vi "Deinitialize Cameras.vi"(8 "error in":errorcluster, 11 "Gantry in":refnum<class "Gantry.lvclass">) -> (0 "error out":errorcluster, 3 "Gantry out":refnum<class "Gantry.lvclass">)   [LabVIEW 2017, in "Gantry.lvclass"]
uses:
  Gantry.lvclass
  FlexWorktable/FlexWorktable.lvclass
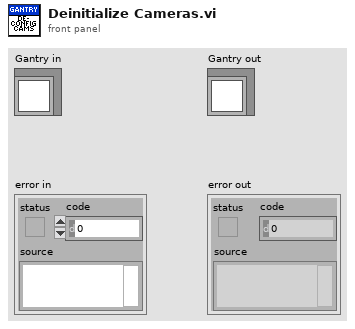
[diagram p1: front panel]
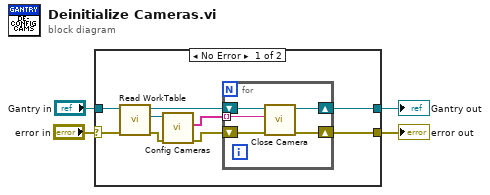
[diagram p0: block diagram]
diagram:
  n1 = case shown="No Error" "error in" {
    selector: "error in" -> [w10 w20]
    tunnel: [w12 w20] -> w3
    tunnel: [w13 w19] -> w1
    tunnel: "Gantry in" -> [w11 w19]
    frame No Error {
      n2 = call-dynamic "Read WorkTable.vi"("error in"=w10, "Gantry Class in"=w11) -> ("error out"=w7:errorcluster, "Worktable"=w9:refnum<class "FlexWorktable.lvclass">, "Gantry Class out"=w8:refnum<class "Gantry.lvclass">)  [unwired: 7 in]
      n3 = call "Config Cameras.vi"("error in (no error)"=w7, "FlexWorktable in"=w9) -> ("error out"=w5:errorcluster, "Array"=w6:string[])  [unwired: 7 in, 1 out]
      n4 = for {
        tunnel: w6 -> [w18] mode=indexing
        shift-right: [w14] -> w12
        shift-left: w5 -> [w15]
        shift-right: [w16] -> w13
        shift-left: w8 -> [w17]
        n5 = call-dynamic "Close Camera.vi"("error in"=w15, "Camera Name"=w18, "Gantry in"=w17) -> ("error out"=w14:errorcluster, "Gantry out"=w16:refnum<class "Gantry.lvclass">)  [unwired: 7 in]
      }
    }
    frame Error {
    }
  }
  "error out" <- w3
  "Gantry out" <- w1
